vi "DAQcardStorage.vi"(2 "error in":errorcluster, 3 "DAQ Card/Channels":i32[](array[numeric]), 4 "Card Settings":T1[](array[typedef]) {"Global Edge Type" items=["Rising"=10280, "Falling"=10171]; "Sample Rate" format="%#_3p"}, 5 "Tree DVR In":refnum<data-value>) -> (0 "error out":errorcluster)   [LabVIEW 2014]
doc: "Stores the 'DAQ' card-wide settings to MDS+"
uses:
  <vilib>/MDSplus/Classes/Tree_Class/Tree.lvclass
  Controls/DigitizerSettingsCardSettings.ctl
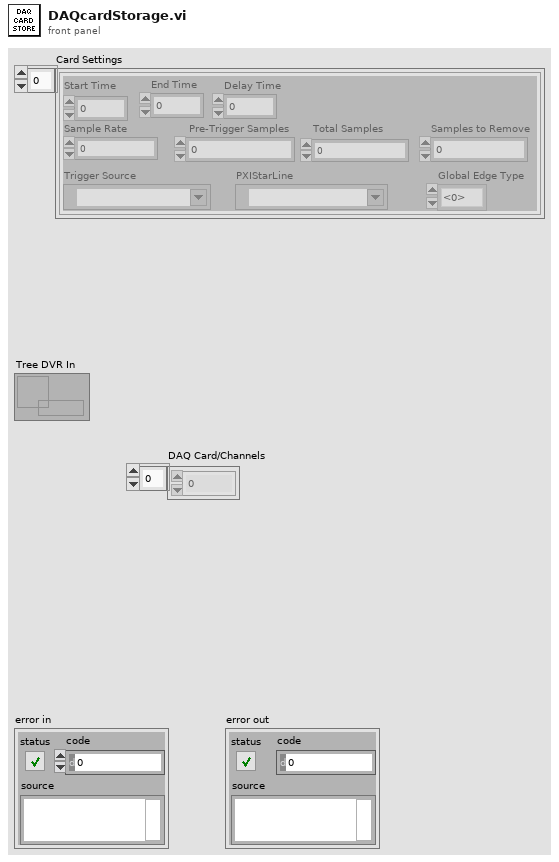
[diagram p1: front panel]
types:
  T1 = typedef "DigitizerSettingsCardSettings.ctl" = cluster{"Start Time":dbl, "End Time":dbl, "Sample Rate":dbl, " Pre-Trigger Samples":u32, "Total Samples":i32, "Samples to Remove":u32, "Trigger Source":tag, "Global Edge Type":i32, "PXIStarLine":tag, "Delay Time":dbl}
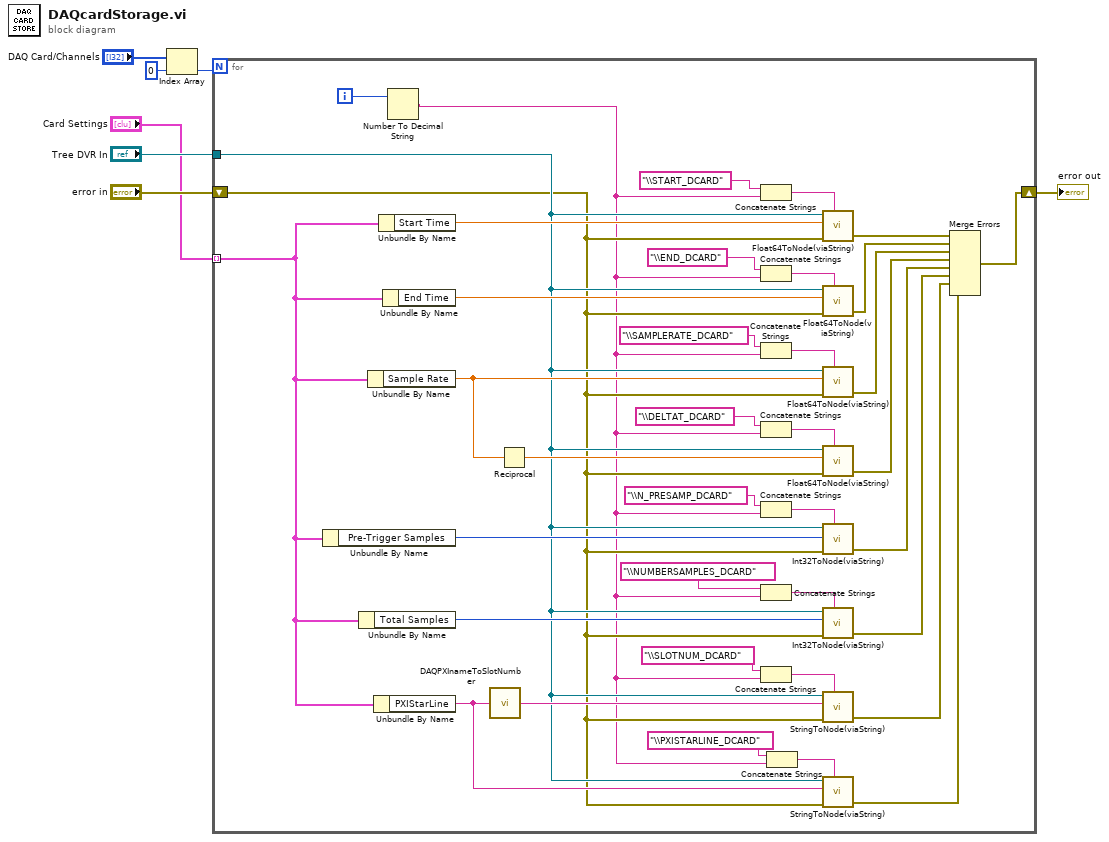
[diagram p0: block diagram]
diagram:
  n1 = Index Array(array="DAQ Card/Channels", index=0) -> (element=w3:i32)
  n2 = for {
    N: w3 -> [_]
    tunnel: "Card Settings" -> [w45] mode=indexing
    tunnel: "Tree DVR In" -> [w14]
    shift-right: [w23] -> w5
    shift-left: "error in" -> [w13]
    i -> [w9]
    n3 = Unbundle By Name(w45) -> ("Pre-Trigger Samples"=w35:u32)
    n4 = Unbundle By Name(w45) -> ("Total Samples"=w33:i32)
    n5 = Unbundle By Name(w45) -> ("Sample Rate"=w37:dbl)
    n6 = Unbundle By Name(w45) -> ("PXIStarLine"=w15:tag)
    n7 = Unbundle By Name(w45) -> ("Start Time"=w43:dbl)
    n8 = Unbundle By Name(w45) -> ("End Time"=w41:dbl)
    n9 = Number To Decimal String(number=w9) -> (decimal integer string=w8:string)  [unwired: 1 in]
    n10 = call "DAQPXInameToSlotNumber.vi"("PXI name"=w15) -> ("Slot #"=w24:string)
    n11 = Reciprocal(x=w37) -> (1/x=w38:dbl)
    n12 = Concatenate Strings("\\START_DCARD" ("string"), w8) -> (w44:string)
    n13 = Concatenate Strings("\\END_DCARD" ("string"), w8) -> (w42:string)
    n14 = Concatenate Strings("\\SAMPLERATE_DCARD" ("string"), w8) -> (w40:string)
    n15 = Concatenate Strings("\\DELTAT_DCARD" ("string"), w8) -> (w39:string)
    n16 = Concatenate Strings("\\N_PRESAMP_DCARD" ("string"), w8) -> (w36:string)
    n17 = Concatenate Strings("\\NUMBERSAMPLES_DCARD" ("string"), w8) -> (w34:string)
    n18 = Concatenate Strings("\\SLOTNUM_DCARD" ("string"), w8) -> (w32:string)
    n19 = Concatenate Strings("\\PXISTARLINE_DCARD" ("string"), w8) -> (w11:string)
    n20 = call "Float64ToNode(viaString).vi"("Tree DVR in"=w14, "DBL in"=w43, "error in"=w13, "NodePath"=w44) -> ("error out"=w31:errorcluster)  [unwired: 3 in]
    n21 = call "Float64ToNode(viaString).vi"("Tree DVR in"=w14, "DBL in"=w41, "error in"=w13, "NodePath"=w42) -> ("error out"=w30:errorcluster)  [unwired: 3 in]
    n22 = call "Float64ToNode(viaString).vi"("Tree DVR in"=w14, "DBL in"=w37, "error in"=w13, "NodePath"=w40) -> ("error out"=w29:errorcluster)  [unwired: 3 in]
    n23 = call "Float64ToNode(viaString).vi"("Tree DVR in"=w14, "DBL in"=w38, "error in"=w13, "NodePath"=w39) -> ("error out"=w28:errorcluster)  [unwired: 3 in]
    n24 = call "Int32ToNode(viaString).vi"("Tree DVR in"=w14, "I32 in"=w35, "error in (no error)"=w13, "NodePath"=w36) -> ("error out"=w27:errorcluster)  [unwired: 3 in]
    n25 = call "Int32ToNode(viaString).vi"("Tree DVR in"=w14, "I32 in"=w33, "error in (no error)"=w13, "NodePath"=w34) -> ("error out"=w26:errorcluster)  [unwired: 3 in]
    n26 = call "StringToNode(viaString).vi"("Tree DVR in"=w14, "String value in"=w24, "error in (no error)"=w13, "NodePath"=w32) -> ("error out"=w25:errorcluster)  [unwired: 3 in]
    n27 = call "StringToNode(viaString).vi"("Tree DVR in"=w14, "String value in"=w15, "error in (no error)"=w13, "NodePath"=w11) -> ("error out"=w10:errorcluster)  [unwired: 3 in]
    n28 = Merge Errors(w31, w30, w29, w28, w27, w26, w25, w10) -> (w23:errorcluster)
  }
  "error out" <- w5
